vi "read position from xml.vi"(8 "error in (no error)":errorcluster, 10 "XML in":string, 11 "Autofocus in":refnum<class "Autofocus.lvclass">) -> (0 "error out":errorcluster, 3 "Autofocus out":refnum<class "Autofocus.lvclass">)   [LabVIEW 2012, in "Autofocus.lvclass"]
uses:
  Autofocus.lvclass
  Autofocus.lvclass/Autofocus.ctl
  <vilib>/Distrio/Murmex/Message/Message.lvclass
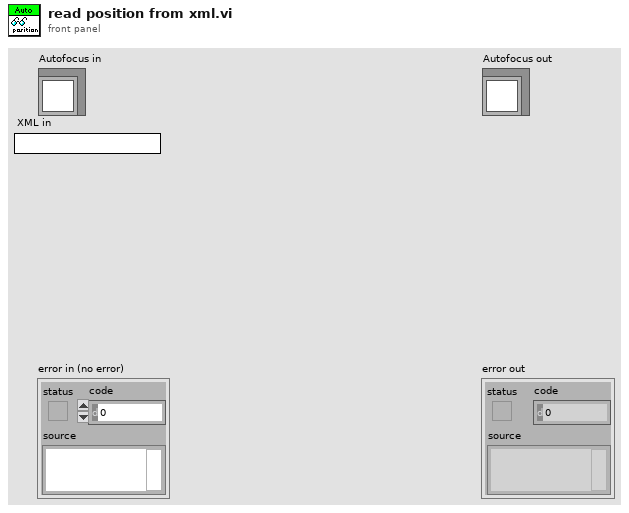
[diagram p1: front panel]
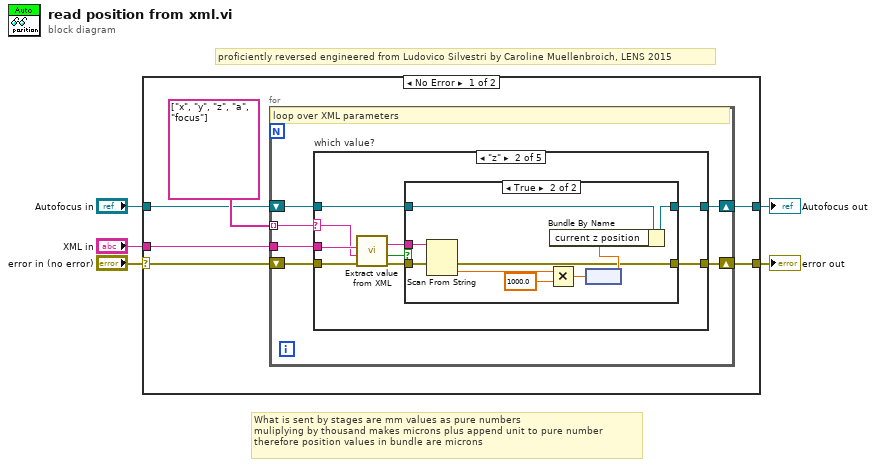
[diagram p0: block diagram]
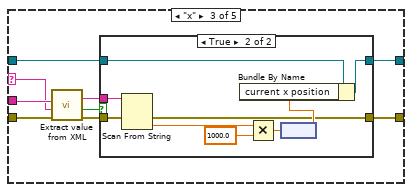
[diagram p4: hidden frame]
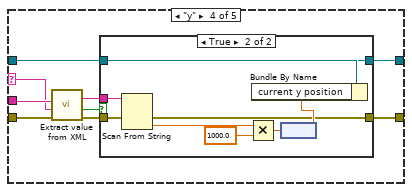
[diagram p6: hidden frame]
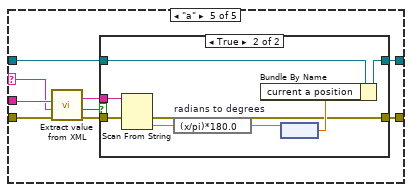
[diagram p8: hidden frame]
diagram:
  # "proficiently reversed engineered from Ludovico Silvestri by Caroline Muellenbroich, LENS 2015"
  # "What is sent by stages are mm values as pure numbers\nmuliplying by thousand makes microns plus append unit to pure number\ntherefore position values in bundle are microns"
  n1 = case shown="No Error" "error in (no error)" {
    selector: "error in (no error)" -> [w8 w100]
    tunnel: [w7 w100] -> w4
    tunnel: [w9 w99] -> w2
    tunnel: "Autofocus in" -> [w10 w99]
    tunnel: "XML in" -> [w6 _]
    frame No Error {
      n2 = for {
        shift-right: [w15] -> w9
        shift-left: w10 -> [w16]
        shift-right: [w13] -> w7
        shift-left: w8 -> [w14]
        tunnel: string[] ["x", "y", "z", "a", "focus"] ("keys") -> [w17] mode=indexing
        tunnel: w6 -> [w12]
        # "loop over XML parameters"
        n3 = case "which value?" shown="\"z\"" w17 {
          selector: w17 -> [_ w22 w42 w62 w82]
          tunnel: w16 -> [w19 w28 w48 w68 w88]
          tunnel: [w19 w27 w47 w67 w87] -> w15
          tunnel: w14 -> [w18 w25 w45 w65 w85]
          tunnel: [w18 w26 w46 w66 w86] -> w13
          tunnel: w12 -> [_ w23 w43 w63 w83]
          frame Default {
          }
          frame "z" {
            n4 = call <vilib>:"Extract value from XML.vi"("error in (no error)"=w25, "tag name"=w22, "parameters XML"=w23) -> ("error out"=w24:errorcluster, "found?"=w21:bool, "value"=w20:string)  [unwired: 5 in, 1 out]
            n5 = case shown="True" w21 {
              tunnel: w28 -> [w30 w39]
              tunnel: [w30 w38] -> w27
              tunnel: [w29 w36] -> w26
              tunnel: w24 -> [w29 w35]
              tunnel: w20 -> [_ w34]
              frame False {
              }
              frame True {
                n6 = Scan From String(input string=w34, error in=w35) -> (error out=w36:errorcluster, output 1=w33:dbl)  [unwired: 3 in, 2 out]
                n7 = Multiply(x=w33, y=1000.0) -> (x*y=w32:dbl)
                n8 = node(w32) -> (w37:dbl[unit])
                n9 = Bundle By Name(cluster=w39, "current z position"=w37) -> (w38:refnum<class "Autofocus.lvclass">)
              }
            }
          }
          frame "x" {
            n10 = call <vilib>:"Extract value from XML.vi"("error in (no error)"=w45, "tag name"=w42, "parameters XML"=w43) -> ("error out"=w44:errorcluster, "found?"=w41:bool, "value"=w40:string)  [unwired: 5 in, 1 out]
            n11 = case shown="True" w41 {
              tunnel: w48 -> [w50 w59]
              tunnel: [w50 w58] -> w47
              tunnel: [w49 w56] -> w46
              tunnel: w44 -> [w49 w55]
              tunnel: w40 -> [_ w54]
              frame False {
              }
              frame True {
                n12 = Scan From String(input string=w54, error in=w55) -> (error out=w56:errorcluster, output 1=w51:dbl)  [unwired: 3 in, 2 out]
                n13 = Multiply(x=w51, y=1000.0) -> (x*y=w52:dbl)
                n14 = node(w52) -> (w57:dbl[unit])
                n15 = Bundle By Name(cluster=w59, "current x position"=w57) -> (w58:refnum<class "Autofocus.lvclass">)
              }
            }
          }
          frame "y" {
            n16 = call <vilib>:"Extract value from XML.vi"("error in (no error)"=w65, "tag name"=w62, "parameters XML"=w63) -> ("error out"=w64:errorcluster, "found?"=w61:bool, "value"=w60:string)  [unwired: 5 in, 1 out]
            n17 = case shown="True" w61 {
              tunnel: w68 -> [w70 w79]
              tunnel: [w70 w78] -> w67
              tunnel: [w69 w76] -> w66
              tunnel: w64 -> [w69 w75]
              tunnel: w60 -> [_ w74]
              frame False {
              }
              frame True {
                n18 = Scan From String(input string=w74, error in=w75) -> (error out=w76:errorcluster, output 1=w72:dbl)  [unwired: 3 in, 2 out]
                n19 = Multiply(x=w72, y=1000.0) -> (x*y=w71:dbl)
                n20 = node(w71) -> (w77:dbl[unit])
                n21 = Bundle By Name(cluster=w79, "current y position"=w77) -> (w78:refnum<class "Autofocus.lvclass">)
              }
            }
          }
          frame "a" {
            n22 = call <vilib>:"Extract value from XML.vi"("error in (no error)"=w85, "tag name"=w82, "parameters XML"=w83) -> ("error out"=w84:errorcluster, "found?"=w81:bool, "value"=w80:string)  [unwired: 5 in, 1 out]
            n23 = case shown="True" w81 {
              tunnel: w88 -> [w90 w98]
              tunnel: [w90 w97] -> w87
              tunnel: [w89 w95] -> w86
              tunnel: w84 -> [w89 w94]
              tunnel: w80 -> [_ w93]
              frame False {
              }
              frame True {
                n24 = Scan From String(input string=w93, error in=w94) -> (error out=w95:errorcluster, output 1=w91:dbl)  [unwired: 3 in, 2 out]
                n25 = expression code="(x/pi)*180.0" "radians to degrees"(w91) -> (w92:dbl)
                n26 = node(w92) -> (w96:dbl[unit])
                n27 = Bundle By Name(cluster=w98, "current a position"=w96) -> (w97:refnum<class "Autofocus.lvclass">)
              }
            }
          }
        }
      }
    }
    frame Error {
    }
  }
  "error out" <- w4
  "Autofocus out" <- w2
